vi "Initialize.vi"(8 "error in (no error)":errorcluster, 11 "DemoDAQ in":refnum<class "DemoDAQ.lvclass">) -> (0 "error out":errorcluster, 3 "DemoDAQ out":refnum<class "DemoDAQ.lvclass">)   [LabVIEW 2020, in "DemoDAQ.lvlib" / "DemoDAQ.lvclass"]
uses:
  DemoDAQ.lvclass
  DemoDAQ.lvclass/DemoDAQ.ctl
  Hardware Abstraction Layer/Component/DAQ/DAQ/DAQ.lvclass
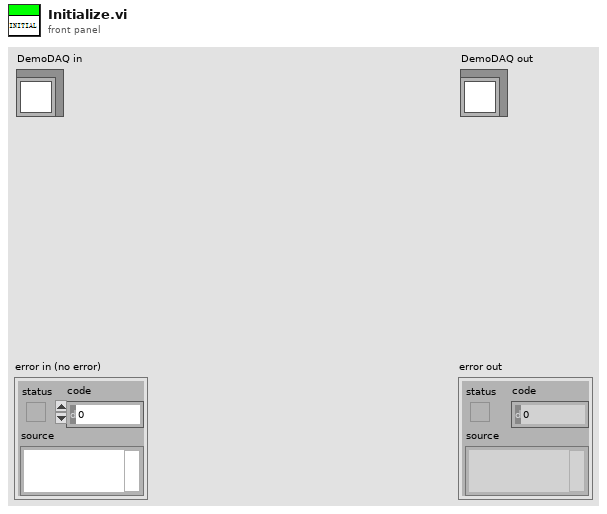
[diagram p1: front panel]
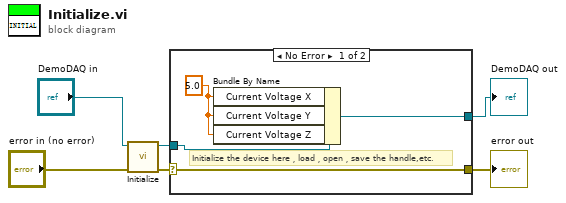
[diagram p0: block diagram]
diagram:
  n1 = call-parent "Initialize.vi"("error in (no error)"="error in (no error)", "DAQ in"="DemoDAQ in") -> ("error out"=w3:errorcluster, "DAQ out"=w4:refnum<class "DemoDAQ.lvclass">)  [unwired: 8 in]
  n2 = case shown="No Error" w3 {
    selector: w3 -> [w9 w12]
    tunnel: [w9 w12] -> w2
    tunnel: [w8 w11] -> w1
    tunnel: w4 -> [w10 w11]
    frame No Error {
      w7 = 5.0 ("Current Voltage Z")
      # "Initialize the device here，load，open，save the handle,etc."
      n3 = Bundle By Name(cluster=w10, "Current Voltage X"=w7, "Current Voltage Y"=w7, "Current Voltage Z"=w7) -> (w8:refnum<class "DemoDAQ.lvclass">)
    }
    frame Error {
    }
  }
  "error out" <- w2
  "DemoDAQ out" <- w1
